vi "CalcAngles.vi"(10 "Widths, um":dbl[](array[numeric]), 11 "Distances, mm":dbl[](array[numeric])) -> (3 "Angles, mrad":dbl[](array[numeric]))   [LabVIEW 2017]
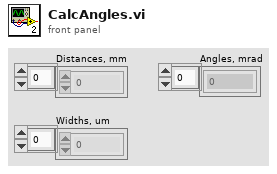
[diagram p1: front panel]
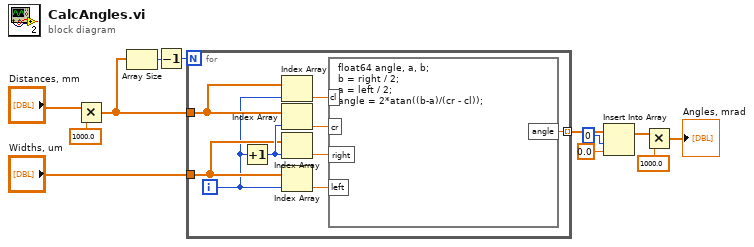
[diagram p0: block diagram]
diagram:
  n1 = Multiply(x="Distances, mm", y=1000.0) -> (x*y=w4:dbl[])
  n2 = Array Size(array=w4) -> (size(s)=w10:i32)
  n3 = Decrement(x=w10) -> (x-1=w11:i32)
  n4 = for {
    N: w11 -> [_]
    tunnel: w4 -> [w16]
    tunnel: "Widths, um" -> [w20]
    tunnel: [w13] -> w9 mode=indexing
    i -> [w15]
    n5 = Increment(x=w15) -> (x+1=w21:i32)
    n6 = Index Array(array=w16, index=w15) -> (element=w14:dbl)
    n7 = Index Array(array=w16, index=w21) -> (element=w19:dbl)
    n8 = Index Array(array=w20, index=w21) -> (element=w18:dbl)
    n9 = Index Array(array=w20, index=w15) -> (element=w17:dbl)
    n10 = formula code="float64 angle, a, b;\nb = right / 2;\na = left / 2;\nangle = 2*atan((b-a)/(cr - cl));"("cr"=w19, "right"=w18, "left"=w17, "cl"=w14) -> ("angle"=w13:dbl)
  }
  n11 = Insert Into Array(array=w9, index=0, new element=0.0 ("new element/subarray")) -> (w3:dbl[])
  n12 = Multiply(x=w3, y=1000.0) -> (x*y=→"Angles, mrad":dbl[])
